vi "Reset.vi"(8 "error in (no error)":errorcluster, 11 "Progress in":refnum<class "Progress.lvclass">) -> (0 "error out":errorcluster, 3 "Progress out":refnum<class "Progress.lvclass">)   [LabVIEW 2021, in "Progress.lvlib" / "Progress.lvclass"]
uses:
  Progress.lvclass
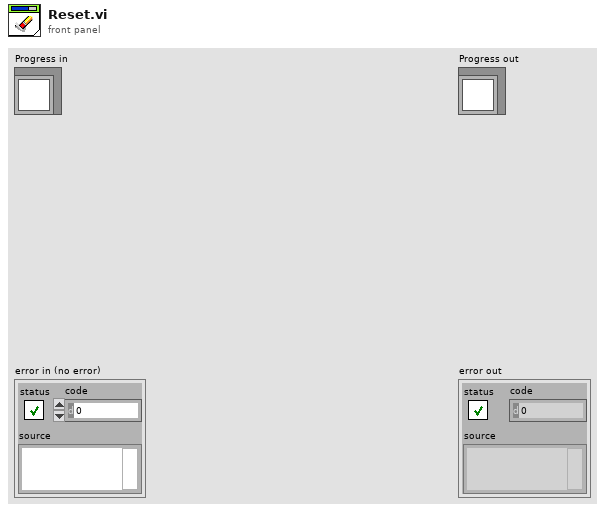
[diagram p1: front panel]
types:
  T1 = typedef "Progress.lvlib/Progress.lvclass/Data.ctl" = cluster{"SlideRefnum":refnum<vi>, "ProgressValue":u64, "NbElement":u64, "Caption":string, "UINotifier":refnum<notifier>, "StopUI":refnum<user-event>}
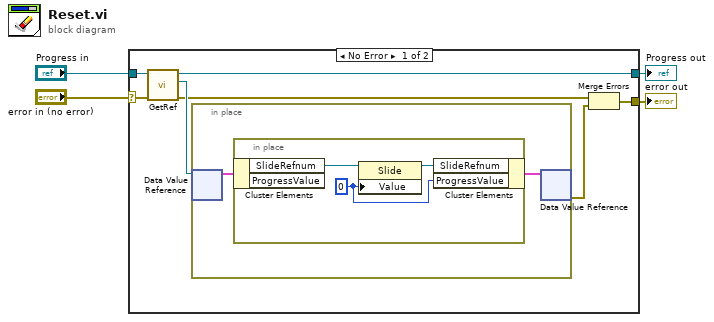
[diagram p0: block diagram]
diagram:
  n1 = case shown="No Error" "error in (no error)" {
    selector: "error in (no error)" -> [w8 w18]
    tunnel: [w5 w18] -> w3
    tunnel: [w9 w17] -> w1
    tunnel: "Progress in" -> [w11 w17]
    frame No Error {
      n2 = call "GetRef.vi"("error in (no error)"=w8, "Progress in"=w11) -> ("error out"=w6:errorcluster, "ref"=w10:refnum<data-value>, "Progress out"=w9:refnum<class "Progress.lvclass">)  [unwired: 7 in]
      n3 = in-place {
        n4 = in-place-dvr #1(w10) -> (w13:T1)  [unwired: 1 out]
        n5 = in-place {
          w14 = u64 0
          n6 = in-place-cluster #2(w13) -> ("SlideRefnum"=w16:refnum<vi>)  [unwired: 1 out]
          n7 = property class="Slide"(reference=w16, "Value"=w14) -> (reference out=w15:refnum<vi>)  [unwired: 1 in, 1 out]
          n8 = in-place-cluster #2("SlideRefnum"=w15, "ProgressValue"=w14) -> (w12:T1)
        }
        n9 = in-place-dvr #1(w12) -> (w7:errorcluster)  [unwired: 1 out]
      }
      n10 = Merge Errors(w6, w7) -> (w5:errorcluster)
    }
    frame Error {
    }
  }
  "error out" <- w3
  "Progress out" <- w1
